vi "Init.vi"(10 "Setup":T1) -> (3 "Base Setup out":refnum<class "Base Setup.lvclass">)   [LabVIEW 2025, in "jettl.lvlib" / "Setup.lvlib" / "Base Setup.lvclass"]
uses:
  Base Setup.lvclass
  Setup.ctl
  Attributes/Attributes/Attributes.lvclass
  Transport/Transport/Transport.lvclass
  Refs/Refs.lvclass
  Msg Set.ctl
  Msg/Msg.lvclass
  Actor/Actor.lvclass
  Base Setup.lvclass/Base Setup.ctl
  jettl.lvlib
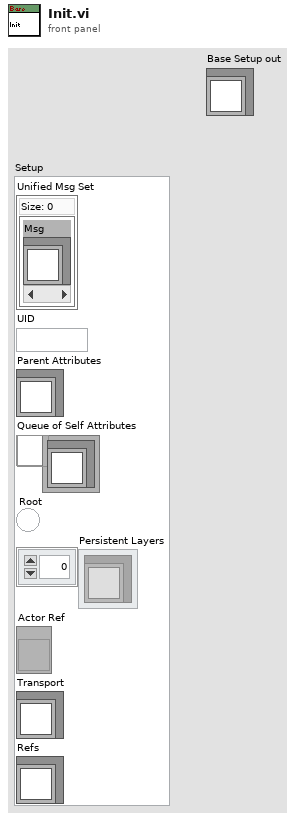
[diagram p1: front panel]
types:
  T1 = typedef "jettl.lvlib/Setup.ctl" = cluster{"Unified Msg Set":T2, "UID":string, "Parent Attributes":refnum<class "Attributes.lvclass">, "Queue of Self Attributes":refnum<queue>, "Root":bool, "Persistent Layers":refnum<class "Actor.lvclass">[], "Actor Ref":refnum<vi>, "Transport":refnum<class "Transport.lvclass">, "Refs":refnum<class "Refs.lvclass">}
  T2 = typedef "jettl.lvlib/Msg Set.ctl" = set{refnum<class "Msg.lvclass">}
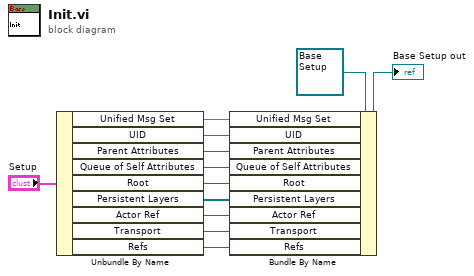
[diagram p0: block diagram]
diagram:
  n1 = Unbundle By Name("Setup") -> ("Unified Msg Set"=w9:T2, "UID"=w8:string, "Parent Attributes"=w7:refnum<class "Attributes.lvclass">, "Queue of Self Attributes"=w6:refnum<queue>, "Root"=w5:bool, "Persistent Layers"=w4:refnum<class "Actor.lvclass">[], "Actor Ref"=w3:refnum<vi>, "Transport"=w2:refnum<class "Transport.lvclass">, "Refs"=w1:refnum<class "Refs.lvclass">)
  n2 = Bundle By Name(cluster=refnum<class "Base Setup.lvclass"> refnum ("Base Setup out"), "Unified Msg Set"=w9, "UID"=w8, "Parent Attributes"=w7, "Queue of Self Attributes"=w6, "Root"=w5, "Persistent Layers"=w4, "Actor Ref"=w3, "Transport"=w2, "Refs"=w1) -> (→"Base Setup out":refnum<class "Base Setup.lvclass">)
